vi "Party Time Drive Too.vi"   [LabVIEW 2018]
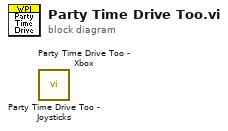
[diagram p0: block diagram]
diagram:
  n1 = call "Party Time Drive Too - Joysticks.vi"() -> ()  [unwired: 10 in, 2 out]
  n2 = call "Party Time Drive Too - Xbox.vi"() -> ()  [unwired: 10 in, 2 out]
